vi "Draw PDO Slots.vi"(8 "error in":errorcluster, 9 "PDO Mappable Entries":refnum<class "OD Entry.lvclass">[](array[class]), 10 "PDO Slots":refnum<class "PDO Slot.lvclass">[](array[class]), 11 "PDO Grid in":refnum<class "PDO Grid.lvclass">) -> (0 "error out":errorcluster, 3 "PDO Grid out":refnum<class "PDO Grid.lvclass">)   [LabVIEW 2020, in "PDO Grid.lvlib" / "PDO Grid.lvclass"]
uses:
  PDO Grid.lvclass
  D:/git/Sourcegrid-LabVIEW/source/Grid/SourceGrid.lvclass
  PDO Slot/PDO Slot.lvclass
  Core/OD Entry/OD Entry.lvclass
  Core/OD Sub-Entry/OD Sub-Entry.lvclass
  D:/git/EDS-File-Viewer/source/Core/OD Entry/OD Entry.lvclass
  Sourcegrid-LabVIEW/source/Grid/SourceGrid.lvclass
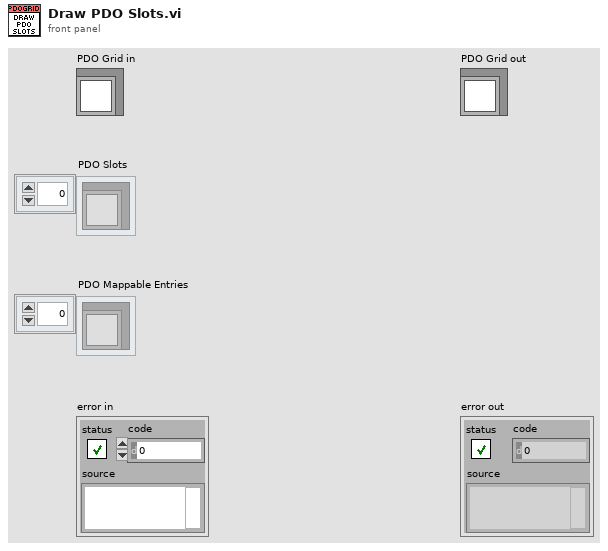
[diagram p1: front panel]
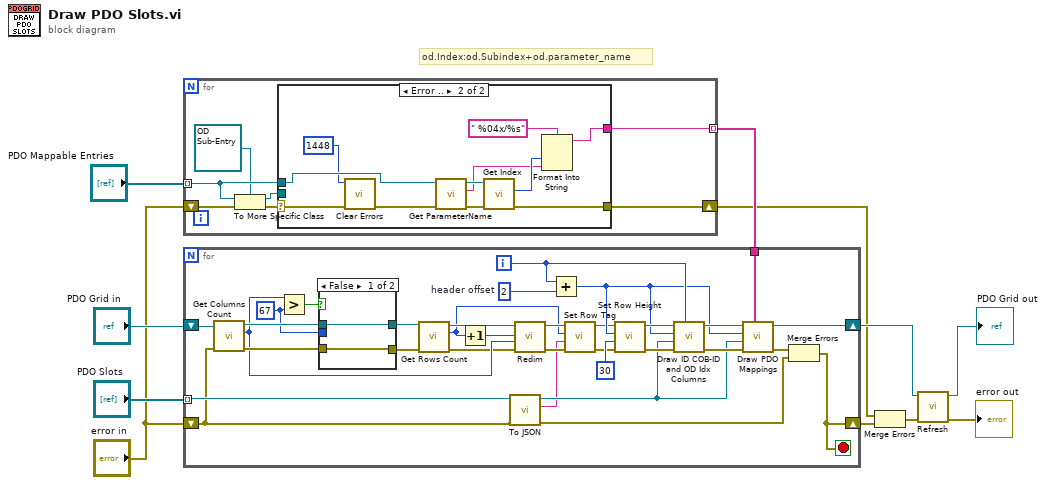
[diagram p0: block diagram]
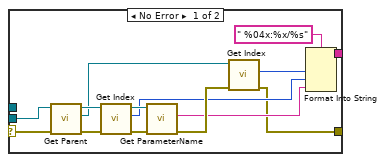
[diagram p2: hidden frame]
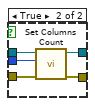
[diagram p3: hidden frame]
diagram:
  # "od.Index:od.Subindex+od.parameter_name"
  n1 = for {
    tunnel: "PDO Mappable Entries" -> [w18] mode=indexing
    shift-right: [w14] -> w2
    shift-left: "error in" -> [w15]
    tunnel: [w13] -> w4 mode=indexing
    n2 = To More Specific Class(target class=refnum<class "OD Sub-Entry.lvclass"> refnum ("Electronic Datasheet.lvlib:OD Sub-Entry"), reference=w18, error in=w15) -> (specific class reference=w12:refnum<class "OD Sub-Entry.lvclass">, error out=w16:errorcluster)
    n3 = case shown="Error .." w16 {
      selector: w16 -> [w32 w38]
      tunnel: w18 -> [_ w43]
      tunnel: [w20 w36] -> w14
      tunnel: [w19 w35] -> w13
      tunnel: w12 -> [w30 _]
      frame No Error {
        n4 = call "Get Parent.vi"("Error In"=w32, "reference in"=w30) -> ("Error Out"=w28:errorcluster, "Parent"=w29:refnum<class "OD Entry.lvclass">, "reference out"=w31:refnum<class "OD Sub-Entry.lvclass">)  [unwired: 7 in]
        n5 = call "Get Index.vi"("Error In"=w28, "reference in"=w31) -> ("Error Out"=w27:errorcluster, "Index"=w22:u16, "reference out"=w25:refnum<class "OD Sub-Entry.lvclass">)  [unwired: 7 in]
        n6 = call "Get ParameterName.vi"("Error In"=w27, "reference in"=w25) -> ("Error Out"=w26:errorcluster, "ParameterName"=w21:string)  [unwired: 7 in, 1 out]
        n7 = call "Get Index.vi"("Error In"=w26, "reference in"=w29) -> ("Error Out"=w20:errorcluster, "Index"=w23:u16)  [unwired: 7 in, 1 out]
        n8 = Format Into String(format string=" %04x:%x/%s", w23, w22, w21) -> (resulting string=w19:string)  [unwired: 2 in, 1 out]
      }
      frame Error {
        n9 = call <vilib>:"Clear Errors.vi"("error in (no error)"=w38, "specific error code to clear (0: all)"=1448) -> ("error out"=w34:errorcluster)  [unwired: 4 in, 1 out]
        n10 = call "Get ParameterName.vi"("Error In"=w34, "reference in"=w43) -> ("Error Out"=w39:errorcluster, "ParameterName"=w37:string, "reference out"=w40:refnum<class "OD Entry.lvclass">)  [unwired: 7 in]
        n11 = call "Get Index.vi"("Error In"=w39, "reference in"=w40) -> ("Error Out"=w36:errorcluster, "Index"=w42:u16)  [unwired: 7 in, 1 out]
        n12 = Format Into String(format string=" %04x/%s", w42, w37) -> (resulting string=w35:string)  [unwired: 2 in, 1 out]
      }
    }
  }
  n13 = for {
    tunnel: "PDO Slots" -> [w56] mode=indexing
    shift-right: [w45] -> w9
    shift-left: "error in" -> [w46]
    shift-right: [w57] -> w7
    shift-left: "PDO Grid in" -> [w76]
    tunnel: w4 -> [w53]
    i -> [w60]
    stop <- w45 stop-if-true
    w64 = 2  # header offset
    w72 = 67 ("x")
    n14 = call "Get Columns Count.vi"("error in"=w46, "SourceGrid in"=w76) -> ("error out"=w73:errorcluster, "Columns Count"=w70:i32, "SourceGrid out"=w74:refnum<class "PDO Grid.lvclass">)  [unwired: 7 in]
    n15 = Greater?(x=w70, y=w72) -> (0:w75:bool)
    n16 = case shown="False" w75 {
      tunnel: w74 -> [w78 w82]
      tunnel: w73 -> [w77 w83]
      tunnel: w72 -> [_ w81]
      tunnel: [w78 w80] -> w68
      tunnel: [w77 w79] -> w71
      frame False {
      }
      frame True {
        n17 = call "Set Columns Count.vi"("error in"=w83, "ColumnsCount"=w81, "SourceGrid in"=w82) -> ("error out"=w79:errorcluster, "SourceGrid out"=w80:refnum<class "PDO Grid.lvclass">)  [unwired: 7 in]
      }
    }
    n18 = call "Get Rows Count.vi"("error in"=w71, "SourceGrid in"=w68) -> ("error out"=w69:errorcluster, "Rows Count"=w49:i32, "SourceGrid out"=w67:refnum<class "PDO Grid.lvclass">)  [unwired: 7 in]
    n19 = Increment(x=w49) -> (x+1=w66:i32)
    n20 = call "To JSON.vi"("error in"=w46, "PDO Slot in"=w56) -> ("error out"=w44:errorcluster, "JSON"=w47:string, "PDO Slot out"=w48:refnum<class "PDO Slot.lvclass">)  [unwired: 7 in]
    n21 = call "Redim.vi"("error in"=w69, "Columns"=w70, "Rows"=w66, "Sourcegrid in"=w67) -> ("error out"=w65:errorcluster, "Sourcegrid out"=w51:refnum<class "PDO Grid.lvclass">)  [unwired: 6 in]
    n22 = Add(x=w60, y=w64) -> (x+y=w55:i32)
    n23 = call "Set Row Tag.vi"("error in"=w65, "object"=w47, "Row Index"=w49, "SourceGrid in"=w51) -> ("error out"=w52:errorcluster, "SourceGrid out"=w50:refnum<class "PDO Grid.lvclass">)  [unwired: 6 in]
    n24 = call "Set Row Height.vi"("error in"=w52, "Height"=30, "Row"=w55, "SourceGrid in"=w50) -> ("error out"=w62:errorcluster, "SourceGrid out"=w61:refnum<class "PDO Grid.lvclass">)  [unwired: 6 in]
    n25 = call "Draw ID COB-ID and OD Idx Columns.vi"("PDO Slot Index"=w60, "error in"=w62, "PDO Slot in"=w48, "Row"=w55, "PDO Grid in"=w61) -> ("error out"=w54:errorcluster, "PDO Grid out"=w58:refnum<class "PDO Grid.lvclass">)  [unwired: 5 in]
    n26 = call "Draw PDO Mappings.vi"("PDO Mappables"=w53, "error in"=w54, "PDO Slot in"=w48, "Row"=w55, "PDO Grid in"=w58) -> ("error out"=w59:errorcluster, "PDO Grid out"=w57:refnum<class "PDO Grid.lvclass">)  [unwired: 5 in]
    n27 = Merge Errors(w59, w44) -> (w45:errorcluster)
  }
  n28 = Merge Errors(w2, w9) -> (w3:errorcluster)
  n29 = call "Refresh.vi"("error in"=w3, "SourceGrid in"=w7) -> ("error out"=→"error out":errorcluster, "SourceGrid out"=→"PDO Grid out":refnum<class "PDO Grid.lvclass">)  [unwired: 8 in]
